vi "Decision for inst wo step (SubVI).vi"(10 "Write channel parameters":dbl[](array[numeric]), 11 "Precision":dbl) -> (1 "Rate":dbl, 2 "Present value":dbl, 3 "Target":dbl, 4 "Sweep required?":bool, 5 "Factor":dbl)   [LabVIEW 2025]
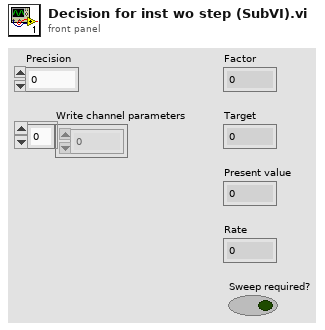
[diagram p1: front panel]
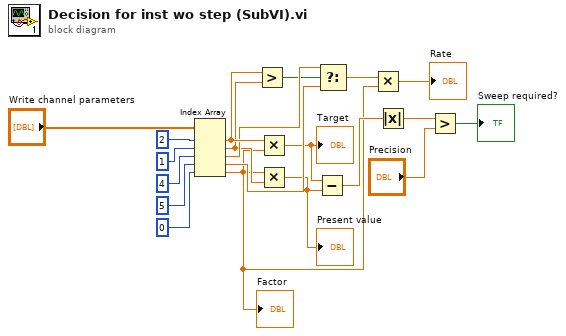
[diagram p0: block diagram]
diagram:
  n1 = Index Array(array="Write channel parameters", index #1=2 ("index"), index #2=1 ("index"), index #3=4 ("index"), index #4=5 ("index"), index #5=0 ("index")) -> (element #1=w19:dbl, element #2=w4:dbl, element #3=w11:dbl, element #4=w12:dbl, element #5=w3:dbl)
  "Factor" <- w3
  n2 = Greater?(x=w19, y=w4) -> (0:w10:bool)
  n3 = Multiply(x=w19, y=w3) -> (x*y=w1:dbl)
  "Target" <- w1
  n4 = Multiply(x=w3, y=w4) -> (x*y=w2:dbl)
  "Present value" <- w2
  n5 = Subtract(x=w1, y=w2) -> (x-y=w13:dbl)
  n6 = Select(t=w11, s=w10, f=w12) -> (s? t:f=w17:dbl)
  n7 = Multiply(x=w17, y=w3) -> (x*y=→"Rate":dbl)
  n8 = Absolute Value(x=w13) -> (abs(x)=w14:dbl)
  n9 = Greater?(x=w14, y="Precision") -> (0:→"Sweep required?":bool)
